vi "Unique Numbers and Multiplicity (DBL).vi"(11 "Numbers":dbl[](array[numeric]) format="%#.6g") -> (0 "error":i32, 2 "Multiplicity":u32[](array[numeric]), 3 "Unique Numbers":dbl[](array[numeric]) format="%#.6g")   [LabVIEW 2014, in "NI_AALPro.lvlib"]
doc: "Obtains all the unique numbers from the input array and determines the multiplicity of each unique number. Wire data to the <B>Numbers</B> input to determine the polymorphic instance to use or manually select the instance."
uses:
  NI_AALPro.lvlib
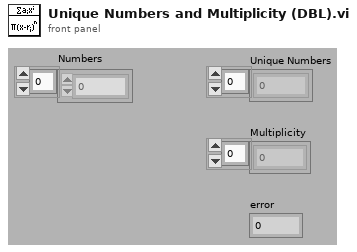
[diagram p1: front panel]
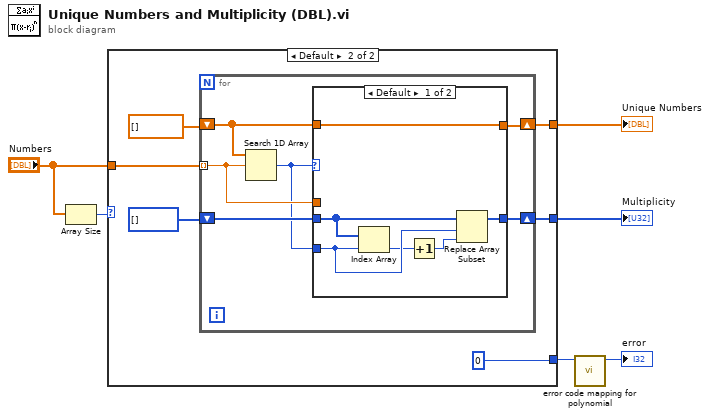
[diagram p0: block diagram]
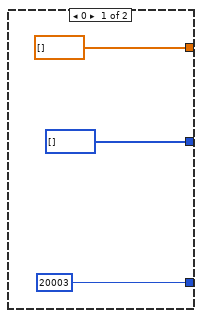
[diagram p2: hidden frame]
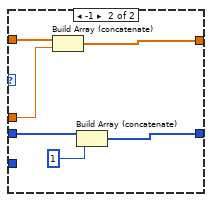
[diagram p3: hidden frame]
diagram:
  n1 = Array Size(array="Numbers") -> (size(s)=w4:i32)
  n2 = case shown="Default" w4 {
    tunnel: "Numbers" -> [_ w15]
    tunnel: [dbl[] [] w12] -> w6
    tunnel: [u32[] [] w11] -> w5
    tunnel: [20003 ("empty array") 0] -> w2
    frame 0 {
    }
    frame Default {
      n3 = for {
        tunnel: w15 -> [w20] mode=indexing
        shift-right: [w19] -> w12
        shift-left: dbl[] [] -> [w21]
        shift-right: [w17] -> w11
        shift-left: u32[] [] -> [w18]
        n4 = Search 1D Array(1D array=w21, element=w20) -> (index of element=w16:i32)  [unwired: 1 in]
        n5 = case shown="Default" w16 {
          tunnel: w21 -> [w22 w33]
          tunnel: w20 -> [_ w32]
          tunnel: [w22 w31] -> w19
          tunnel: w18 -> [w24 w30]
          tunnel: [w23 w28] -> w17
          tunnel: w16 -> [w27 _]
          frame Default {
            n6 = Index Array(array=w24, index=w27) -> (element=w26:u32)
            n7 = Increment(x=w26) -> (x+1=w25:u32)
            n8 = Replace Array Subset(array=w24, new element=w25, index=w27) -> (w23:u32[])
          }
          frame -1 {
            n9 = Build Array (concatenate)(w33, w32) -> (w31:dbl[])
            n10 = Build Array (concatenate)(w30, u32 1) -> (w28:u32[])
          }
        }
      }
    }
  }
  "Unique Numbers" <- w6
  "Multiplicity" <- w5
  n11 = call "error code mapping for polynomial.vi"("error in"=w2) -> ("error out"=→"error":i32)  [unwired: 10 in]
